vi "measure_laser_power.vi"() -> ()   [LabVIEW 2023]
uses:
  <vilib>/Utility/file.llb/Write Delimited Spreadsheet (DBL).vi
panel:
  out "Pulse Energy Data":dbl[][](array[numeric])
  out "XY Graph":cluster{dbl[], dbl[]}(graph)
  out "Current Laser Position":dbl
  in  "Averaging Time /s":u32
  out "Power Reading / J":dbl
  in  "stop":bool
  in  "Scan Button":bool
  in  "Final Wavelength / nm":dbl
  in  "Step Size / nm":dbl
  in  "Start Wavelength / nm":dbl
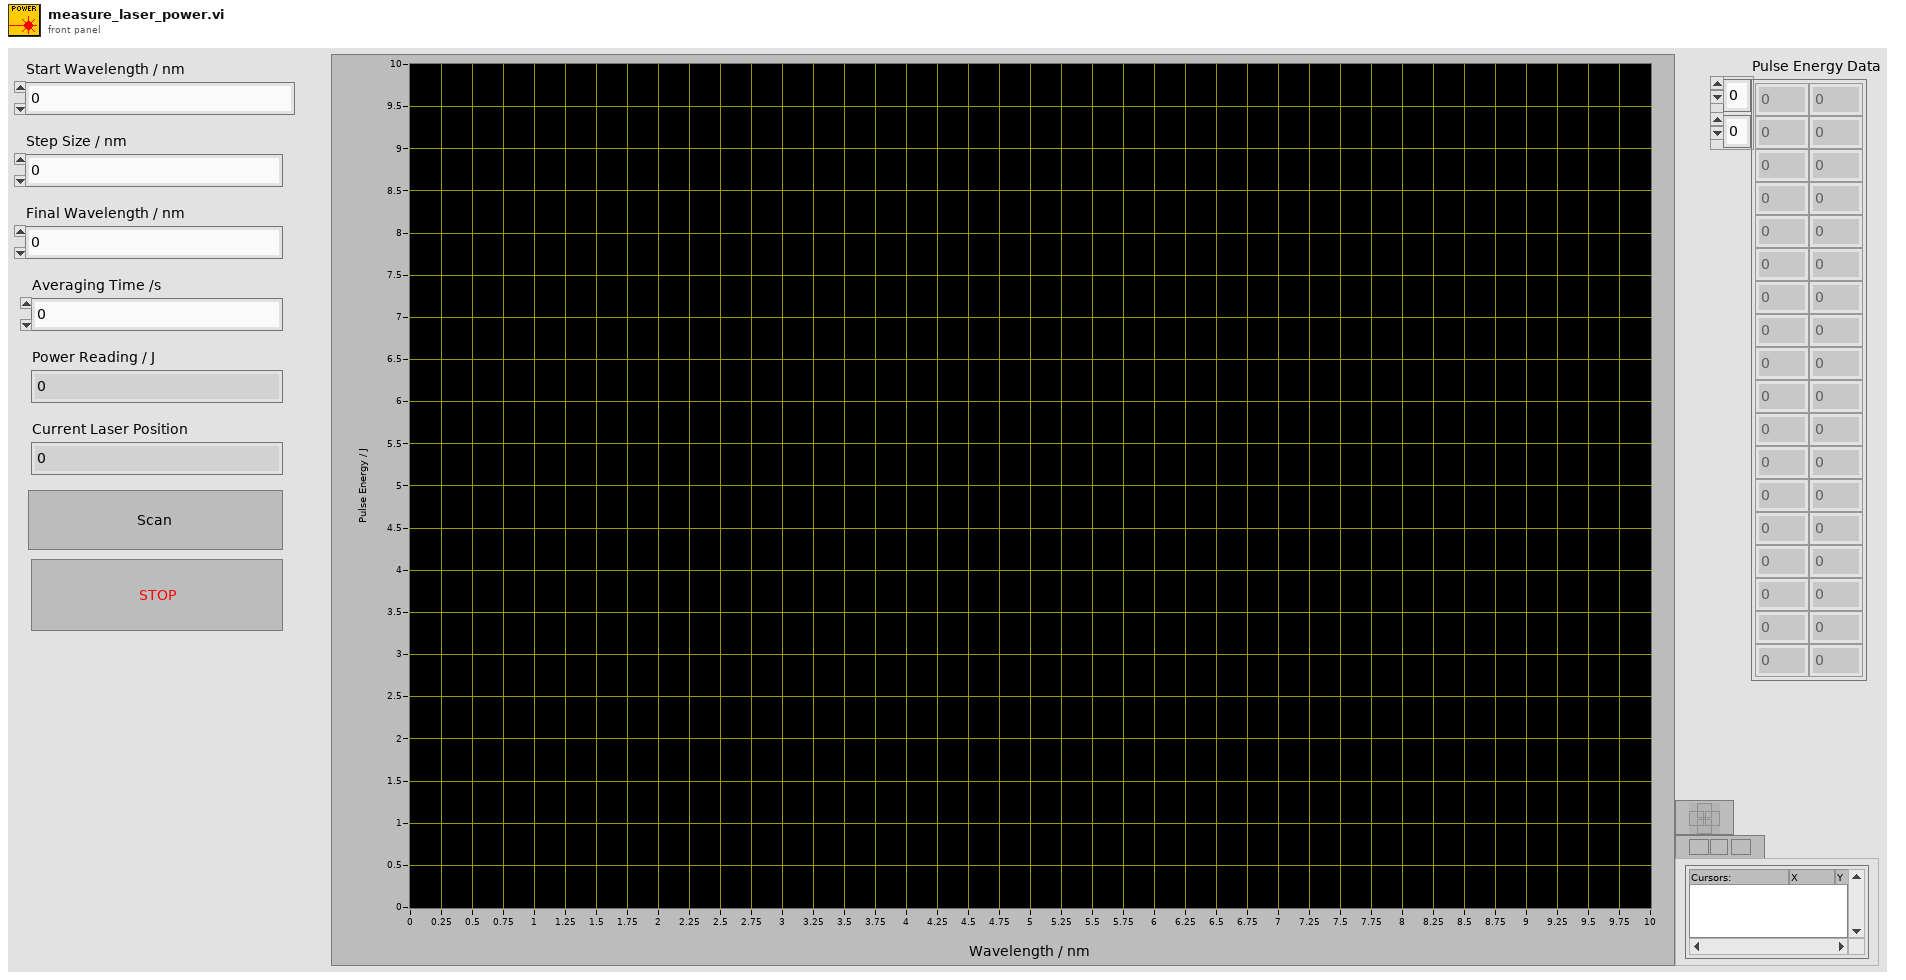
[diagram p1: front panel]
types:
  T1 = cluster{"queue out":refnum<queue>, "error out":errorcluster}
  T2 = cluster{"OphirLMMeasurementLib.ICoLMMeasurement2":refnum<k7>, "Error":errorcluster, "hDevice":i32}
  T3 = cluster{"notifier out":refnum<notifier>, "error out":errorcluster}
  T4 = cluster{"Power Reading ":dbl, "T imestamp":dbl, "Status":i32}
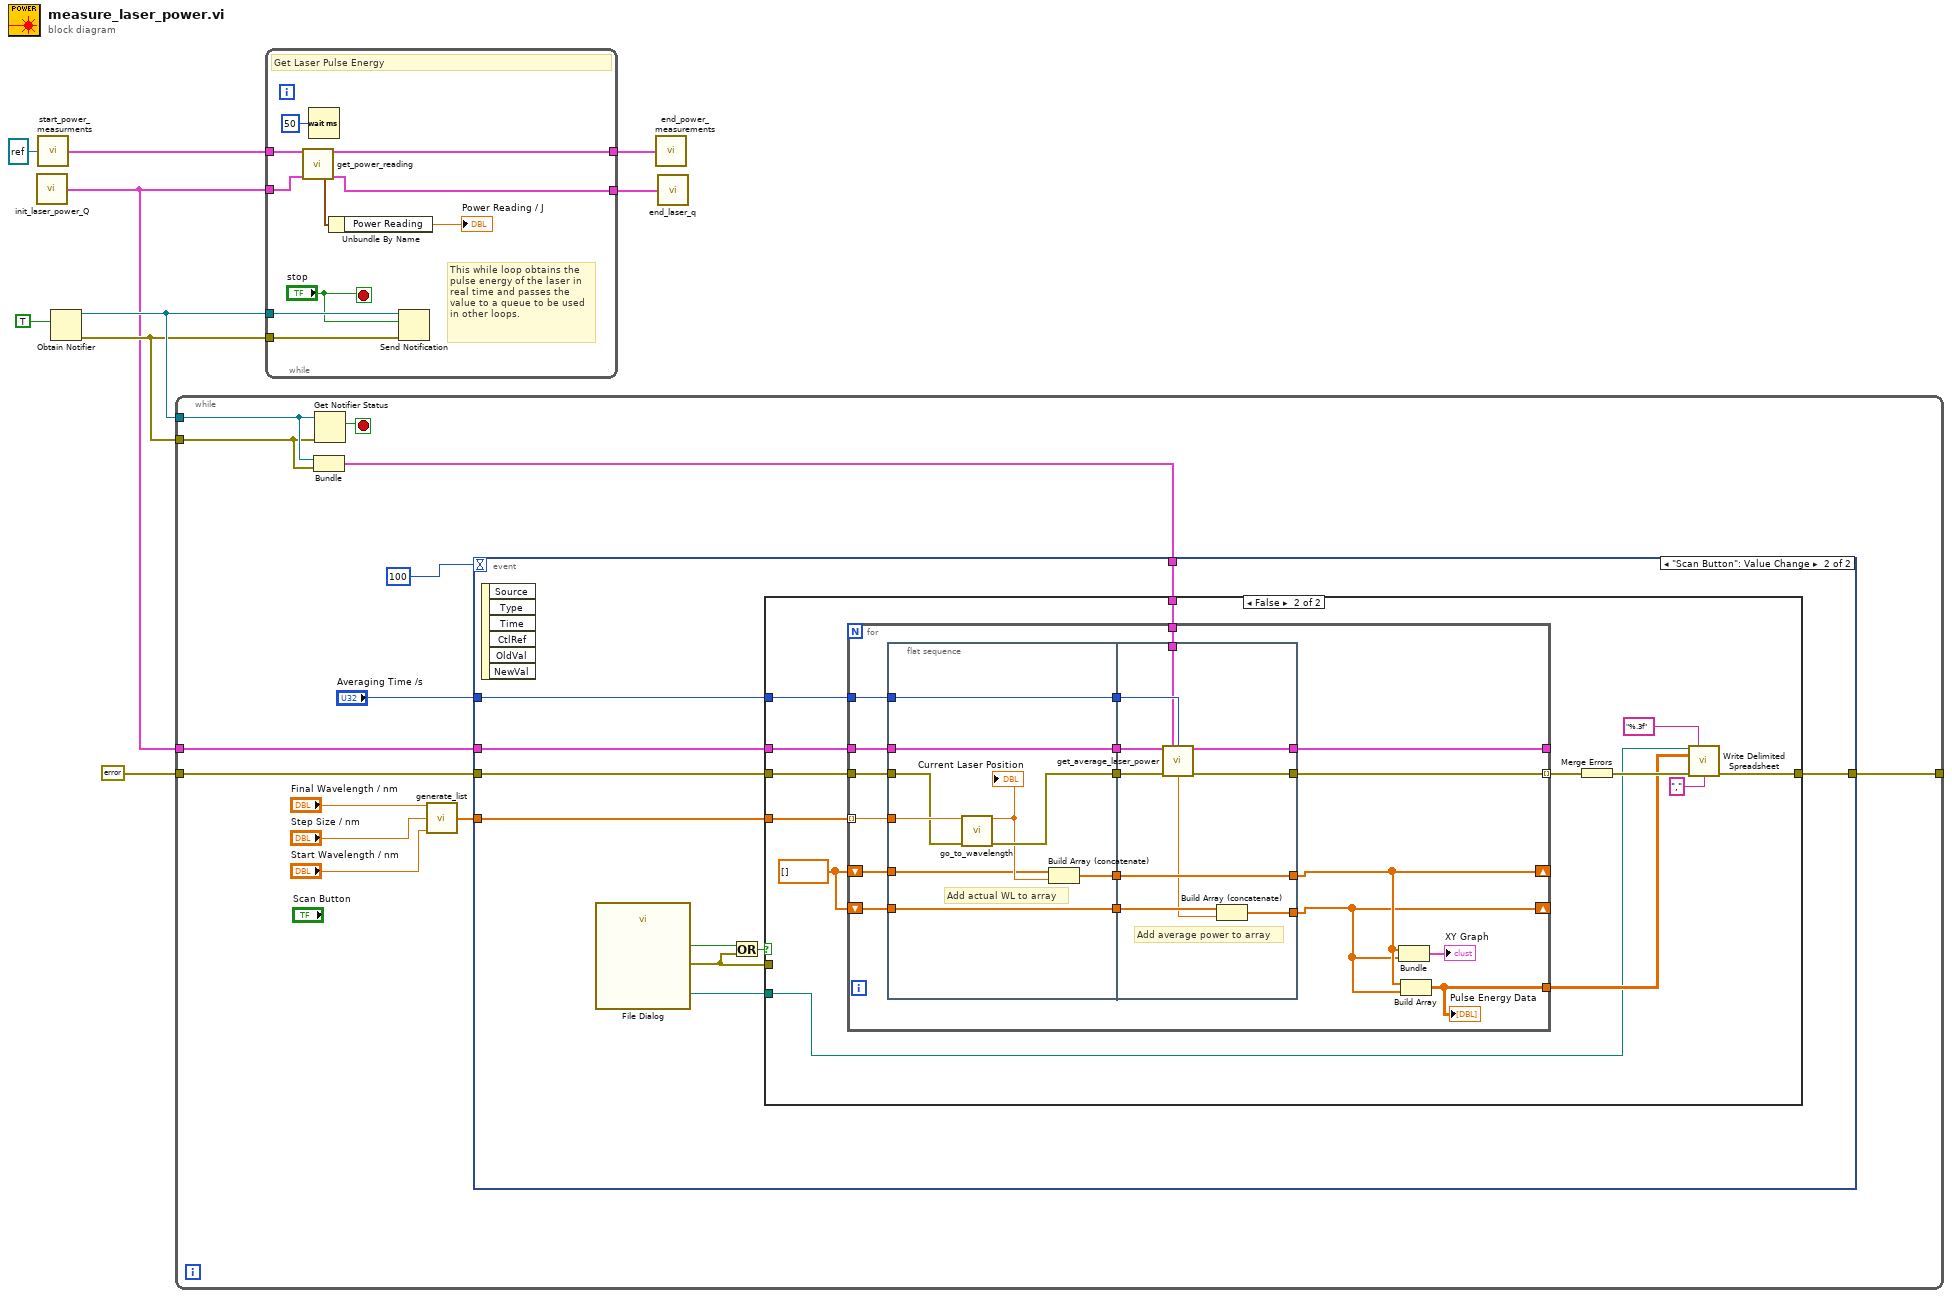
[diagram p0: block diagram]
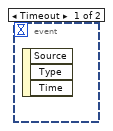
[diagram p2: hidden frame]
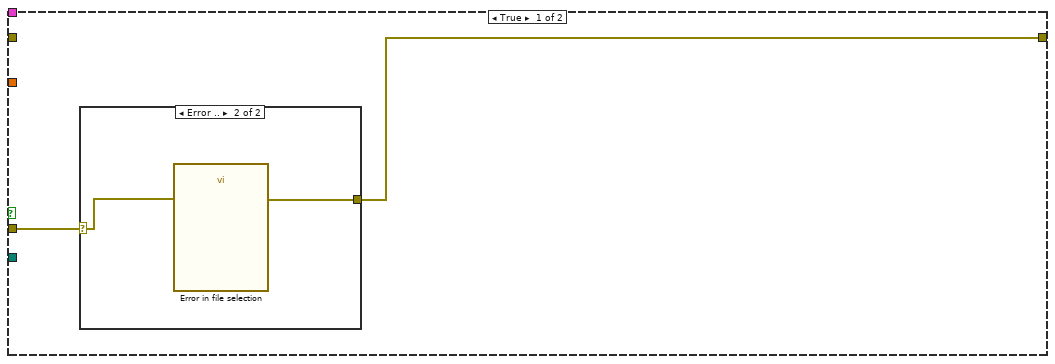
[diagram p3: hidden frame]
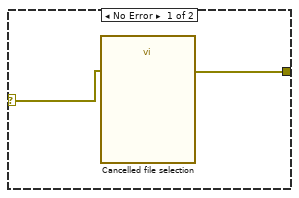
[diagram p4: hidden frame]
diagram:
  n1 = call "init_laser_power_Q.vi"() -> ("Laser Power Q"=w2:T1)  [unwired: 15 in]
  n2 = call "start_power_measurments.vi"("OphirLMMeasurementLib.ICoLMMeasurement2"=refnum<k7> refnum) -> ("Power Meter Connection Data Out"=w9:T2)  [unwired: 14 in]
  n3 = Obtain Notifier(notification data type=TRUE) -> (notifier out=w4:refnum<notifier>, error out=w3:errorcluster)  [unwired: 3 in, 1 out]
  n4 = while {
    tunnel: w4 -> [w13]
    tunnel: w3 -> [w12]
    tunnel: w2 -> [w16]
    tunnel: errorcluster {"status"=FALSE, "code"=0, "source"=""} ("Error in") -> [w15]
    tunnel: [w10] -> _
    stop <- w17 stop-if-true
    n5 = Bundle("notifier out"=w13, "error out"=w12) -> (w11:T3)  [unwired: 1 in]
    n6 = Get Notifier Status(notifier=w13, error in (no error)=w12) -> (current notification=w17:bool)  [unwired: 4 out]
    n7 = call "generate_list.vi"("Upper bound"="Final Wavelength / nm", "Step Size"="Step Size / nm", "Lower Bound"="Start Wavelength / nm") -> ("Array"=w18:dbl[])  [unwired: 12 in]
    n8 = event shown="[1] \"Scan Button\": Value Change" {
      selector: _ -> [_ _]
      dyn-events: _ -> [_ _]
      timeout: 100 -> [_ _]
      tunnel: w18 -> [_ w32]
      tunnel: w16 -> [_ w31]
      tunnel: w15 -> [_ w30]
      tunnel: [_ w29] -> w10
      tunnel: "Averaging Time /s" -> [_ w28]
      tunnel: w11 -> [_ w27]
      event Timeout {
        n9 = event-data() -> ()  [unwired: 1 in, 3 out]
      }
      event "Scan Button": Value Change {
        n10 = event-data() -> ()  [unwired: 1 in, 6 out]
        n11 = call "File Dialog"() -> ("selected path"=w23:path, "cancelled"=w26:bool, "error out"=w24:errorcluster)  [unwired: 12 in, 1 out]
        n12 = Or(x=w26, y=w24) -> (x .or. y?=w25:bool)
        n13 = case shown="False" w25 {
          tunnel: w32 -> [_ w51]
          tunnel: w31 -> [_ w50]
          tunnel: w30 -> [_ w49]
          tunnel: [w33 w42] -> w29
          tunnel: w28 -> [_ w47]
          tunnel: w27 -> [_ w45]
          tunnel: w24 -> [w34 _]
          tunnel: w23 -> [_ w40]
          frame True {
            n14 = case shown="Error .." w34 {
              selector: w34 -> [w36 w38]
              tunnel: [w35 w37] -> w33
              frame No Error {
                n15 = call "Cancelled file selection"("error in (no error)"=w36) -> ("error out"=w35:errorcluster)  [unwired: 9 in, 1 out]
              }
              frame Error {
                n16 = call "Error in file selection"("error in (no error)"=w38) -> ("error out"=w37:errorcluster)  [unwired: 9 in, 1 out]
              }
            }
          }
          frame False {
            w46 = dbl[] []
            n17 = for {
              tunnel: w51 -> [w69] mode=indexing
              tunnel: w50 -> [w68]
              tunnel: w49 -> [w65]
              tunnel: [w64] -> _
              tunnel: [w63] -> w48 mode=indexing
              tunnel: w47 -> [w62]
              tunnel: w45 -> [w56]
              shift-right: [w54] -> _
              shift-left: w46 -> [w60]
              shift-right: [w53] -> _
              shift-left: w46 -> [w58]
              tunnel: [w52] -> w41
              n18 = flat-sequence {
                tunnel: w69 -> [w76]
                tunnel: w68 -> [w78]
                tunnel: [w78] -> w67
                tunnel: [w74] -> w66
                tunnel: w65 -> [w75]
                tunnel: w62 -> [w77]
                tunnel: [w77] -> w61
                tunnel: w60 -> [w72]
                tunnel: [w71] -> w59
                tunnel: w58 -> [w70]
                tunnel: [w70] -> w57
                tunnel: w67 -> [w88]
                tunnel: w66 -> [w87]
                tunnel: [w86] -> w64
                tunnel: [w85] -> w63
                tunnel: w61 -> [w84]
                tunnel: w59 -> [w83]
                tunnel: [w83] -> w54
                tunnel: w57 -> [w82]
                tunnel: [w80] -> w53
                tunnel: w56 -> [w79]
                frame #0 {
                  # "Add actual WL to array"
                  n19 = call "go_to_wavelength.vi"("Set Laser Position"=w76, "error in (no error)"=w75) -> ("Current Laser Position"=w73:dbl, "error out"=w74:errorcluster)  [unwired: 12 in]
                  "Current Laser Position" <- w73
                  n20 = Build Array (concatenate)(w72, w73) -> (w71:dbl[])
                }
                frame #1 {
                  # "Add average power to array"
                  n21 = call "get_average_laser_power.vi"("Laser Power Q"=w88, "Cancel Notifier"=w79, "Averaging Time /s"=w84, "Error in"=w87) -> ("Laser Power Q Out"=w86:T1, "Average Power / J"=w81:dbl, "Error out"=w85:errorcluster)  [unwired: 9 in]
                  n22 = Build Array (concatenate)(w82, w81) -> (w80:dbl[])
                }
              }
              n23 = Bundle(w54, w53) -> (→"XY Graph":cluster{dbl[], dbl[]})  [unwired: 1 in]
              n24 = Build Array(w54, w53) -> (w52:dbl[][])
              "Pulse Energy Data" <- w52
            }
            n25 = Merge Errors(w48) -> (w43:errorcluster)
            n26 = call-poly <vilib>:"Write Delimited Spreadsheet.vi"("file path (dialog if empty)"=w40, "format (%.3f)"="%.3f", "2D data"=w41, "error in (no error)"=w43, "delimiter (\\t)"="," ("delimiter (\\t)")) -> ("error out"=w42:errorcluster)  [unwired: 9 in, 1 out]
          }
        }
      }
    }
  }
  n27 = while {
    tunnel: w2 -> [w97]
    tunnel: w9 -> [w96]
    tunnel: [w95] -> w7
    tunnel: [w94] -> w6
    tunnel: w4 -> [w93]
    tunnel: w3 -> [w92]
    stop <- "stop" stop-if-true
    # "This while loop obtains the pulse energy of the laser in real time and passes the value to a queue to be used in other loops."
    # "Get Laser Pulse Energy"
    n28 = call "get_power_reading.vi"("Power Meter Connection Data In"=w96, "Laser Power Q In"=w97) -> ("Power Meter Connection Data Out"=w95:T2, "Data Out"=w90:T4, "Laser Power Q Out"=w94:T1)  [unwired: 10 in, 1 out]
    n29 = Wait (ms)(milliseconds to wait=u32 50) -> ()  [unwired: 1 out]
    n30 = Unbundle By Name(w90) -> ("Power Reading"=→"Power Reading / J":dbl)
    n31 = Send Notification(notification="stop", notifier=w93, error in (no error)=w92) -> ()  [unwired: 2 out]
  }
  n32 = call "end_power_measurements.vi"("Power Meter Connection Data In"=w7) -> ()  [unwired: 14 in, 1 out]
  n33 = call "end_laser_q.vi"("Laser Power Q In"=w6) -> ()  [unwired: 14 in, 1 out]
